vi "Encapsulate TCP Message.vi"(5 "target_task":string, 6 "source_id":u32, 7 "target_node":u32, 8 "error in (no error)":errorcluster, 9 "type":string, 10 "Encapsulated Msg":refnum<class "Message.lvclass">) -> (0 "error out":errorcluster, 2 "TCP Payload":string)   [LabVIEW 2020, in "Vecto.lvlib"]
uses:
  Vecto.lvlib
  proto/TcpPayload/Data.ctl
  proto/TcpPayload/TcpPayload.lvlib
  SequenceCountService/SequenceCountService.lvclass
  lv-protoc/LV-Proto/Message/Message.lvclass
panel:
  in  "SequenceCountService":refnum<class "SequenceCountService.lvclass">
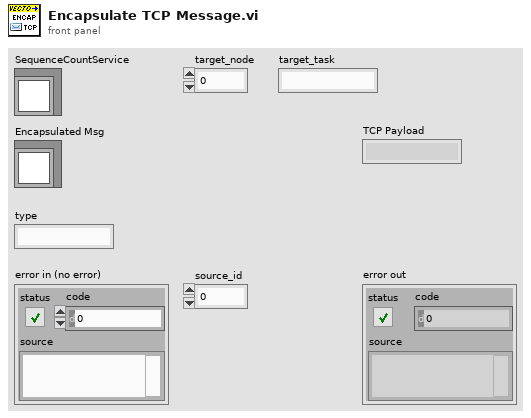
[diagram p1: front panel]
types:
  T1 = typedef "TcpPayload.lvlib/Data.ctl" = cluster{"target_node":u32, "source_id":u32, "sequence":u32, "timestamp":u64, "type":string, "task_id":string, "payload":u8[]}
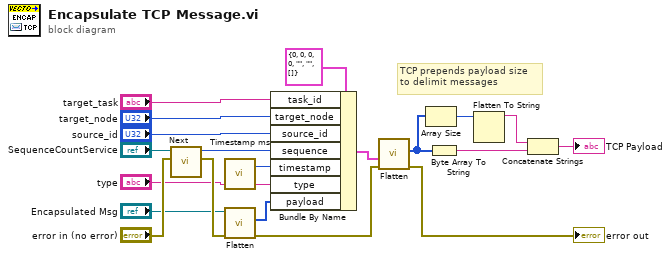
[diagram p0: block diagram]
diagram:
  # "TCP prepends payload size to delimit messages"
  n1 = call "Next.vi"("error in (no error)"="error in (no error)", "SequenceCountService in"="SequenceCountService") -> ("error out"=w19:errorcluster, "Sequence"=w10:u32)  [unwired: 8 in]
  n2 = call "Timestamp ms.vi"() -> ("Timestamp ms"=w12:u64)  [unwired: 7 in]
  n3 = call-dynamic "Flatten.vi"("error in (no error)"=w19, "Message in"="Encapsulated Msg") -> ("error out"=w8:errorcluster, "Buffer"=w13:u8[])  [unwired: 7 in, 1 out]
  n4 = Bundle By Name(cluster=T1 {"target_node"=0, "source_id"=0, "sequence"=0, "timestamp"=0, "type"="", "task_id"="", "payload"=[]} ("TcpPayload"), "task_id"="target_task", "target_node"="target_node", "source_id"="source_id", "sequence"=w10, "timestamp"=w12, "type"="type", "payload"=w13) -> (w9:T1)
  n5 = call "Flatten.vi"("error in"=w8, "Data"=w9) -> ("error out"=→"error out":errorcluster, "Buffer"=w5:u8[])  [unwired: 8 in]
  n6 = Array Size(array=w5) -> (size(s)=w4:i32)
  n7 = Byte Array To String(unsigned byte array=w5) -> (string=w6:string)
  n8 = Flatten To String(anything=w4) -> (data string=w2:string)  [unwired: 3 in, 2 out]
  n9 = Concatenate Strings(w2, w6) -> (→"TCP Payload":string)
